vi "Test Not In Process Loop When Cleared.vi"(8 "error in (no error)":errorcluster, 11 "Test Case In":refnum<class "Process Lifecycle Test.lvclass">) -> (0 "error out":errorcluster, 3 "Test Case Out":refnum<class "Process Lifecycle Test.lvclass">)   [LabVIEW 2020, in "Process Lifecycle Test.lvclass"]
uses:
  Process Lifecycle Test.lvclass
  C:/Program Files (x86)/National Instruments/LabVIEW 2020/vi.lib/Astemes/LUnit/Test Case.lvclass
  source/Framework/Process/Process.lvclass
  source/Framework/Process/Process.lvclass/Process.ctl
  <vilib>/Astemes/LUnit/Test Case.lvclass/Test Case.ctl
  source/Framework/Process/Private/SubVIs/Wait for finish.vi
  source/Framework/Process/Private/SubVIs/Set Lifecycle State.vi
  source/Framework/Process/Protected/Messaging/Send Message.vi
  <vilib>/Utility/error.llb/Clear Errors.vi
  <vilib>/Astemes/LUnit/Append Pass Result.vi
  <vilib>/Astemes/LUnit/Append Fail Result.vi
  source/Framework/Process/Private/SubVIs/Handle Debug Data.vi
  <vilib>/Utility/High Resolution Relative Seconds.vi
  <vilib>/Utility/error.llb/Error Cluster From Error Code.vi
  <vilib>/Astemes/LUnit/Test Case.lvclass
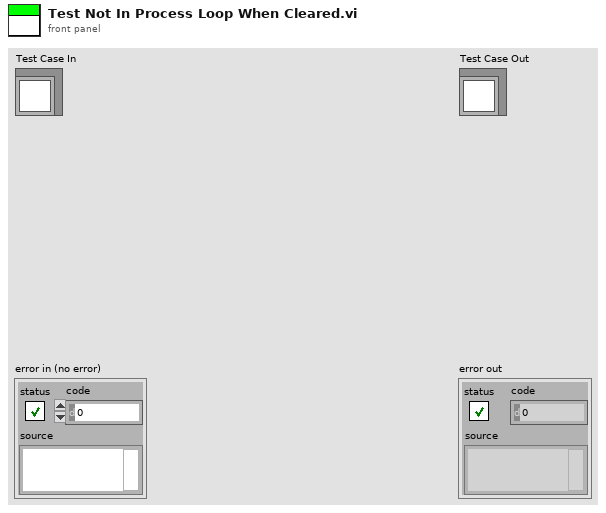
[diagram p1: front panel]
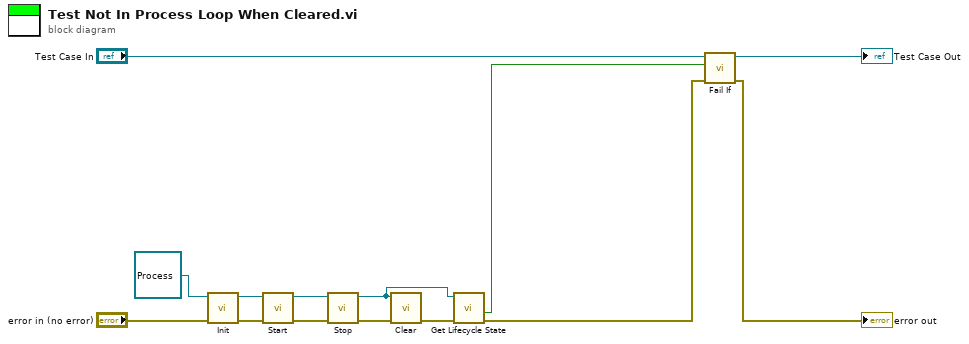
[diagram p0: block diagram]
diagram:
  n1 = call-dynamic "Init.vi"("error in (no error)"="error in (no error)", "Process In"=refnum<class "Process.lvclass"> refnum) -> ("error out"=w8:errorcluster, "Process Out"=w5:refnum<class "Process.lvclass">)  [unwired: 8 in]
  n2 = call "Start.vi"("error in (no error)"=w8, "Process In"=w5) -> ("error out"=w6:errorcluster, "Process Out"=w3:refnum<class "Process.lvclass">)  [unwired: 7 in, 1 out]
  n3 = call "Stop.vi"("error in (no error)"=w6, "Process In"=w3) -> ("error out"=w4:errorcluster, "Process Out"=w1:refnum<class "Process.lvclass">)  [unwired: 7 in, 1 out]
  n4 = call-dynamic "Clear.vi"("error in (no error)"=w4, "Process In"=w1) -> ("error out"=w2:errorcluster)  [unwired: 9 in]
  n5 = call "Get Lifecycle State.vi"("error in (no error)"=w2, "Process In"=w1) -> ("error out"=w10:errorcluster, "In Process Loop?"=w9:bool)  [unwired: 6 in, 2 out]
  n6 = call <vilib>:"Fail If.vi"("error in (no error)"=w10, "Fail?"=w9, "LUnit Test Case In"="Test Case In") -> ("error out"=→"error out":errorcluster, "LUnit Test Case Out"=→"Test Case Out":refnum<class "Process Lifecycle Test.lvclass">)  [unwired: 7 in]
